vi "Memory.Pointer.U8.Read.vi"(8 "error in (no error)":errorcluster, 10 "value":u8, 11 "const U8 Pointer":refnum<class "Memory.Pointer.U8.lvclass">) -> (0 "error out":errorcluster, 2 "value":u8, 3 "U8 Pointer":refnum<class "Memory.Pointer.U8.lvclass">)   [LabVIEW 2016, in "Memory.Pointer.U8.lvclass"]
uses:
  Memory.Pointer.U8.lvclass
  Pointer.Void/Memory.Pointer.Void.lvclass
  C:/Users/Ryan/Documents/Git/Sourcetree/LabVIEW-Memory-Manager/Source/Library/Classes/Pointer/Pointer.Numeric/Memory.Pointer.Numeric.lvclass
  C:/Users/Ryan/Documents/Git/Sourcetree/LabVIEW-Memory-Manager/Source/Library/Classes/Pointer/Pointer.Void/Memory.Pointer.Void.lvclass
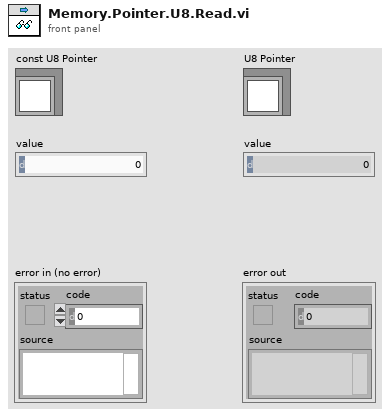
[diagram p1: front panel]
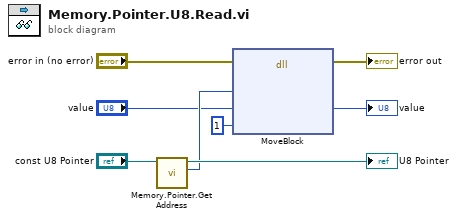
[diagram p0: block diagram]
diagram:
  n1 = call "Memory.Pointer.Get Address.vi"("Pointer in"="const U8 Pointer") -> ("address"=w2:u64, "Pointer out"=→"U8 Pointer":refnum<class "Memory.Pointer.U8.lvclass">)  [unwired: 8 in, 1 out]
  n2 = dll-call lib="LabVIEW" fn="MoveBlock"(error in="error in (no error)", "src"=w2, "dst"="value", "size"=u64 1) -> (error out=→"error out":errorcluster, "dst"=→"value":u8)  [unwired: 5 in, 1 out]
